vi "Wizard Error Handler.vi"(3 "error in":errorcluster) -> (0 "error out":errorcluster)   [LabVIEW 2014]
uses:
  <vilib>/Utility/error.llb/DialogType.ctl
  <vilib>/Utility/file.llb/Read From Spreadsheet File (string).vi
panel:
  out "code out":i32 format="%0.0f"
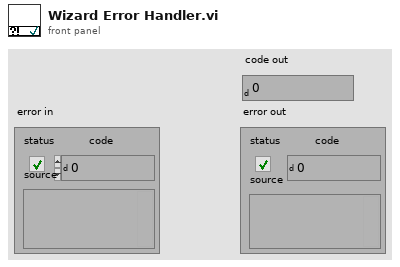
[diagram p1: front panel]
types:
  T1 = typedef "DialogType.ctl" = u16
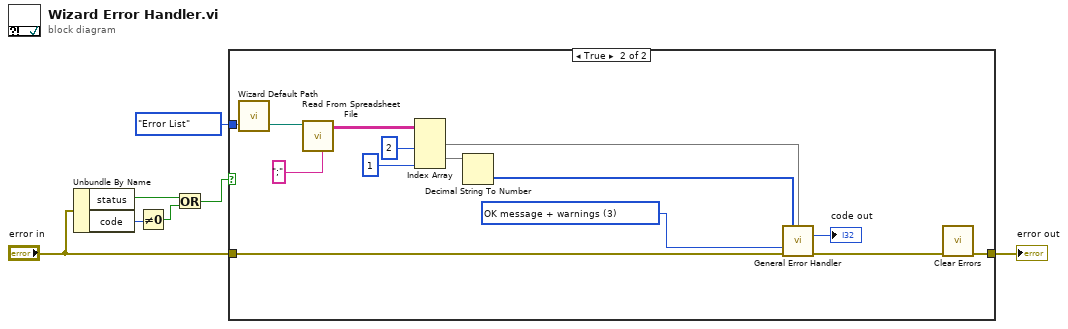
[diagram p0: block diagram]
diagram:
  n1 = Unbundle By Name("error in") -> ("status"=w2:bool, "code"=w4:i32)
  n2 = Not Equal To 0?(x=w4) -> (x != 0?=w3:bool)
  n3 = Or(x=w2, y=w3) -> (x .or. y?=w1:bool)
  n4 = case shown="True" w1 {
    tunnel: enum16{"Error List"}."Error List" ("Mode") -> [_ w22]
    tunnel: [w8 w10] -> w6
    tunnel: "error in" -> [w8 w9]
    frame False {
    }
    frame True {
      w12 = T1 3 items=["no dialog", "OK message", "continue or stop message", "OK message + warnings", "continue/stop + warnings"] ("type of dialog (OK msg:1)")
      n5 = call "Wizard Default Path.vi"("Mode"=w22) -> ("Path"=w21:path)  [unwired: 2 in]
      n6 = call-poly <vilib>:"Read From Spreadsheet File.vi"("delimiter (\\t)"=";" ("delimiter (\\t)"), "file path (dialog if empty)"=w21) -> ("all rows"=w19:string[][])  [unwired: 5 in, 4 out]
      n7 = Index Array(array=w19, index (col) #1=2 ("disabled index (col)"), index (col) #2=1 ("index (col)")) -> (element #1=w16:string[], element #2=w15:string[])  [unwired: 2 in]
      n8 = Decimal String To Number(string=w15) -> (number=w14:i32[])  [unwired: 2 in, 1 out]
      n9 = call <vilib>:"General Error Handler.vi"("[user-defined codes]"=w14, "[user-defined descriptions]"=w16, "type of dialog (OK msg:1)"=w12, "error in (no error)"=w9) -> ("code out"=→"code out":i32, "error out"=w11:errorcluster)  [unwired: 7 in, 3 out]
      n10 = call <vilib>:"Clear Errors.vi"("error in (no error)"=w11) -> ("error out"=w10:errorcluster)  [unwired: 5 in, 1 out]
    }
  }
  "error out" <- w6
